vi "Request Execution Report.vi"(8 "error in (no error)":errorcluster, 10 "Execution":refnum<class "Execution.lvclass">, 11 "Engine in":refnum<class "Engine.lvclass">) -> (0 "error out":errorcluster, 2 "Report":refnum<class "Report.lvclass">, 3 "Engine out":refnum<class "Engine.lvclass">)   [LabVIEW 2020, in "TSnax.lvlib" / "Engine.lvclass"]
uses:
  Engine.lvclass
  Engine.lvclass/Engine.ctl
  Report/Report.lvclass
  Report Response.ctl
  Execution/Execution.lvclass
  Execution Report Request.ctl
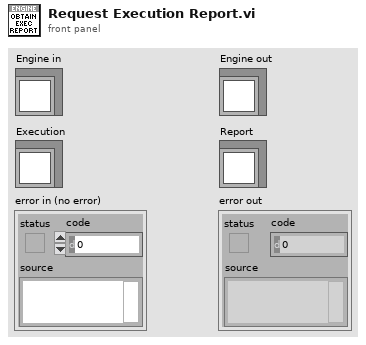
[diagram p1: front panel]
types:
  T1 = typedef "TSnax.lvlib/Engine.lvclass/Execution Report Request.ctl" = cluster{"Execution":refnum<class "Execution.lvclass">, "Notifier":refnum<notifier>}
  T2 = typedef "TSnax.lvlib/Engine.lvclass/Report Response.ctl" = cluster{"Report":refnum<class "Report.lvclass">, "Error":errorcluster}
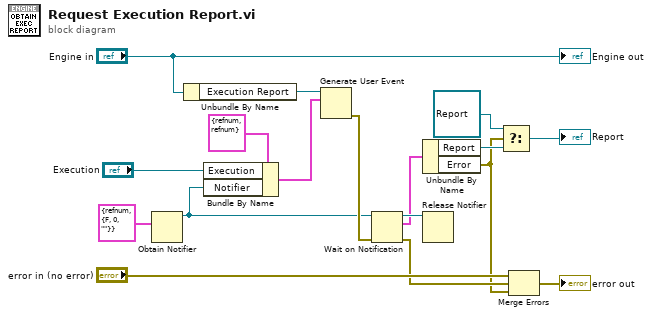
[diagram p0: block diagram]
diagram:
  n1 = Obtain Notifier(notification data type=T2 {"Report"=refnum, "Error"={"status"=FALSE, "code"=0, "source"=""}} ("Report Response")) -> (notifier out=w9:refnum<notifier>)  [unwired: 3 in, 2 out]
  n2 = Unbundle By Name("Engine in") -> ("Execution Report"=w11:refnum<user-event>)
  n3 = Bundle By Name(cluster=T1 {"Execution"=refnum, "Notifier"=refnum} ("Execution Report Request"), "Execution"="Execution", "Notifier"=w9) -> (w10:T1)
  n4 = Generate User Event(user event=w11, event data cluster=w10) -> (error out=w17:errorcluster)  [unwired: 2 in, 1 out]
  n5 = Wait on Notification(notifier=w9, error in (no error)=w17) -> (notifier out=w8:refnum<notifier>, notification=w7:T2, error out=w2:errorcluster)  [unwired: 2 in, 1 out]
  n6 = Unbundle By Name(w7) -> ("Report"=w6:refnum<class "Report.lvclass">, "Error"=w1:errorcluster)
  n7 = Release Notifier(notifier=w8) -> ()  [unwired: 2 in, 3 out]
  n8 = Select(t=refnum<class "Report.lvclass"> refnum, s=w1, f=w6) -> (s? t:f=→"Report":refnum<class "Report.lvclass">)
  n9 = Merge Errors("error in (no error)", w2, w1) -> (→"error out":errorcluster)
  "Engine out" <- "Engine in"
